vi "Set the Internal Project Home.vi"(4 "Error In":errorcluster) -> (0 "Error Out":errorcluster)   [LabVIEW 2014, in "Path Utilities.lvlib"]
uses:
  Path Utilities.lvlib
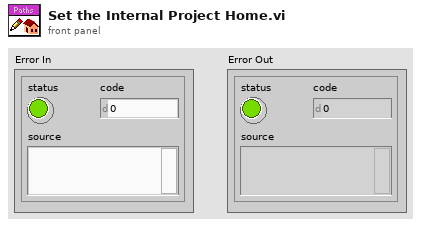
[diagram p1: front panel]
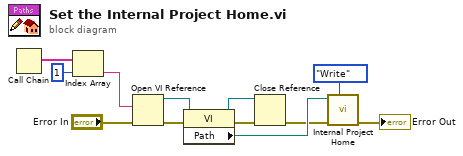
[diagram p0: block diagram]
diagram:
  n1 = Call Chain() -> (call chain=w9:string[])
  n2 = Index Array(array=w9, index=1) -> (element=w6:string)
  n3 = Open VI Reference(vi path=w6, error in (no error)="Error In") -> (vi reference=w4:refnum<vi>, error out=w7:errorcluster)  [unwired: 4 in]
  n4 = property class="VI"(reference=w4, error in=w7) -> (reference out=w1:refnum<vi>, error out=w5:errorcluster, "Path"=w3:path)
  n5 = Close Reference(reference=w1, error in (no error)=w5) -> (error out=w2:errorcluster)
  n6 = call "Internal Project Home.vi"("Function"=enum16{"Read", "Write"}."Write", "Error In"=w2, "Top-Level VI Path"=w3) -> ("Error Out"=→"Error Out":errorcluster)  [unwired: 4 in, 1 out]
